vi "initial.vi"(8 "error in (no error)":errorcluster, 11 "16InOut in":refnum<class "16InOut.lvclass">) -> (0 "error out":errorcluster, 3 "16InOut out":refnum<class "16InOut.lvclass">)   [LabVIEW 2019, in "16InOut.lvclass"]
uses:
  16InOut.lvclass
  C:/Users/user/Desktop/204J1/System/Function/IO Folder/IO_Class/IOCard.lvclass
  IOCard.lvclass/IOCard.ctl
  <vilib>/Instr/_visa.llb/VISA Configure Serial Port (Instr).vi
  IOCard.lvclass
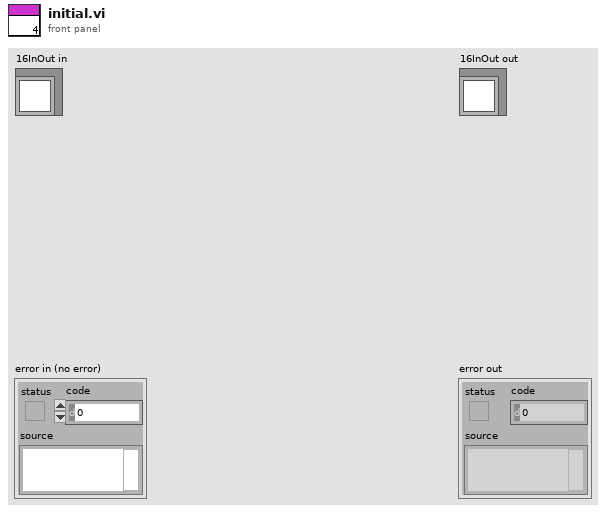
[diagram p1: front panel]
types:
  T1 = cluster{"CardNumber":i32, "Connect":bool, "Handler":i32}
  T2 = typedef "IO Card_Type.ctl" = enum16{"None", "Unidaq32", "6480", "2410C-64", "Zan", "DMC1000B", "16InOut", "Robot", "DMC3600"}
  T3 = cluster{"IO Card Type":T2, "IOType":enum16{"Input", "Output"}, "CardNumber":i32, "ConnectAct":bool, "IP":string}
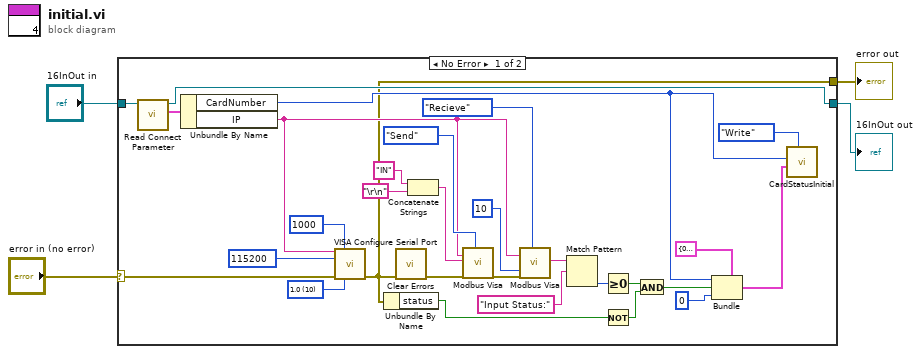
[diagram p0: block diagram]
diagram:
  n1 = case shown="No Error" "error in (no error)" {
    selector: "error in (no error)" -> [w30 w34]
    tunnel: "16InOut in" -> [w33 w35]
    tunnel: [w31 w35] -> w2
    tunnel: [w6 w34] -> w1
    frame No Error {
      w21 = u16 10 items=["1.0"=10, "1.5"=15, "2.0"=20] ("stop bits (10: 1 bit)")
      n2 = call "Read Connect Parameter.vi"("IOCard in"=w33) -> ("Connect Parameter"=w32:T3, "IOCard out"=w31:refnum<class "16InOut.lvclass">)  [unwired: 8 in, 1 out]
      n3 = Unbundle By Name(w32) -> ("CardNumber"=w25:i32, "IP"=w10:string)
      n4 = call-poly "VISA Configure Serial Port"("VISA resource name"=w10, "timeout (10sec)"=u32 1000, "baud rate (9600)"=u32 115200, "error in (no error)"=w30, "stop bits (10: 1 bit)"=w21) -> ("error out"=w6:errorcluster)  [unwired: 9 in, 1 out]
      n5 = Unbundle By Name(w6) -> ("status"=w24:bool)
      n6 = call <vilib>:"Clear Errors.vi"("error in (no error)"=w6) -> ("error out"=w5:errorcluster)  [unwired: 5 in, 1 out]
      n7 = Concatenate Strings("IN" ("Cmd"), "\r\n") -> (w19:string)
      n8 = call "Modbus Visa.vi"("VISA resource name"=w10, "Cmd"=w19, "error in (no error)"=w5, "VisaAction"=enum16{"Open", "Send", "Recieve", "Close"}."Send") -> ("error out"=w17:errorcluster)  [unwired: 14 in, 1 out]
      n9 = call "Modbus Visa.vi"("VISA resource name"=w10, "Time(0.1)"=u32 10, "error in (no error)"=w17, "VisaAction"=enum16{"Open", "Send", "Recieve", "Close"}."Recieve") -> ("read string"=w18:string)  [unwired: 14 in, 1 out]
      n10 = Match Pattern(string=w18, regular expression="Input Status:") -> (offset past match=w20:i32)  [unwired: 1 in, 3 out]
      n11 = Greater Or Equal To 0?(x=w20) -> (x >= 0?=w9:bool)
      n12 = Not(x=w24) -> (.not. x?=w8:bool)
      n13 = And(x=w9, y=w8) -> (x .and. y?=w7:bool)
      n14 = Bundle(cluster=T1 {"CardNumber"=0, "Connect"=FALSE, "Handler"=0} ("DataIn"), "CardNumber"=w25, "Connect"=w7, "Handler"=0) -> (w26:T1)
      n15 = call "CardStatusInitial.vi"("Action"=enum16{"Initial", "Write", "Read", "Release"}."Write", "DataIn"=w26, "CardNumber"=w25) -> ()  [unwired: 8 in, 1 out]
    }
    frame Error {
    }
  }
  "error out" <- w1
  "16InOut out" <- w2
